vi "Variant to MessagePack Object.vi"(8 "error in (no error)":errorcluster, 11 "Input":variant) -> (0 "error out":errorcluster, 3 "msgpack item":u8[](array[numeric]))   [LabVIEW 2020, in "MessagePack.lvlib"]
uses:
  MessagePack.lvlib
  <vilib>/Utility/Data Type/NI_Data Type.lvlib
  635b5c30-cc5e-43b6-8e2f-470f16c0d6f1.vi
  MsgPackString/MsgPackString.lvclass
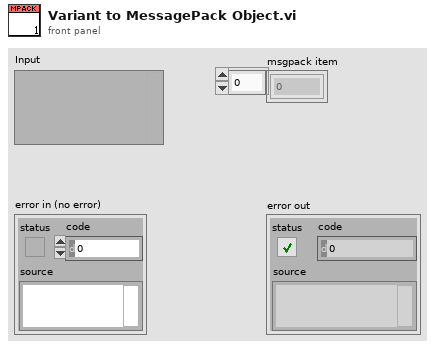
[diagram p1: front panel]
types:
  T1 = typedef "NI_Data Type.lvlib/Data Type.ctl" = enum8{"Invalid Type", "Void", "I8", "I16", "I32", "I64", "U8", "U16", "U32", "U64", "Single Float", "Double Float", "Extended Float", "Single Complex", "Double Complex", "Extended Complex", "Enum U8", "Enum U16", "Enum U32", "Enum U64", "Single Float With Unit", "Double Float With Unit", "Extended Float With Unit", "Single Complex with Unit", "Double Complex with Unit", "Extended Complex with Unit", "Boolean", "String", "Path", "Picture", "Tag", "Array", "Cluster", "Variant", "LV Variant", "Waveform", "Timestamp", "Digital Waveform", "Digital Data", "ExpressData", "Refnum", "External Data", "VI", "Poly VI", "LabVIEW Class Instance", "Fixed Point", "Set Collection", "Map Collection"}
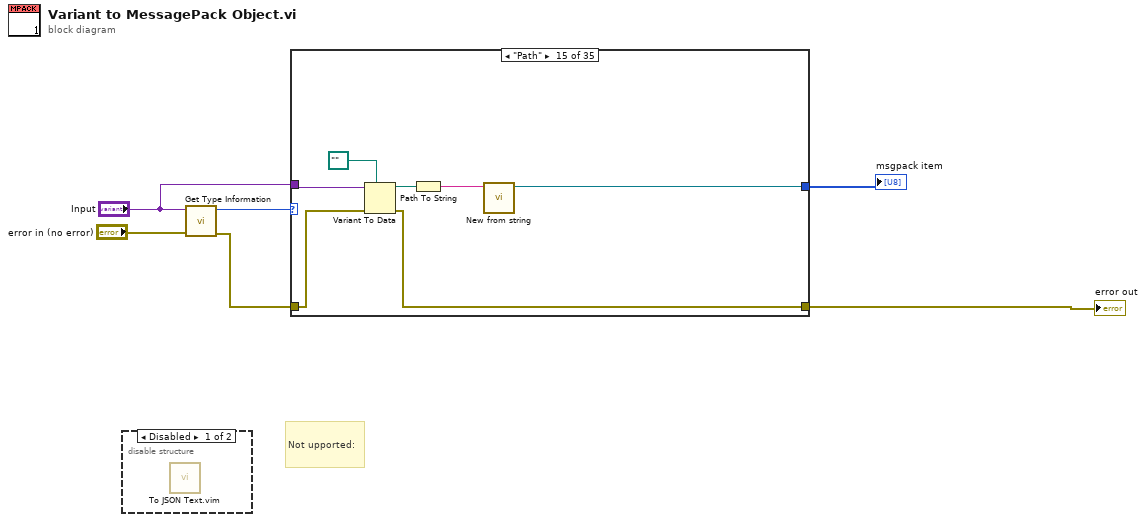
[diagram p0: block diagram]
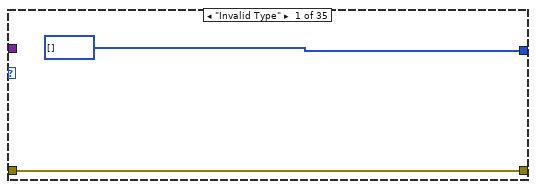
[diagram p3: hidden frame]
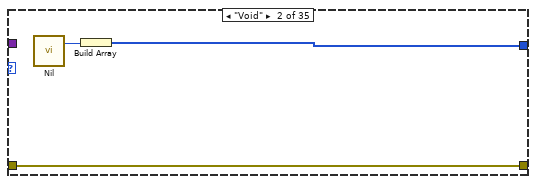
[diagram p4: hidden frame]
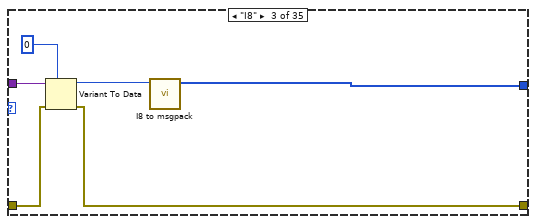
[diagram p5: hidden frame]
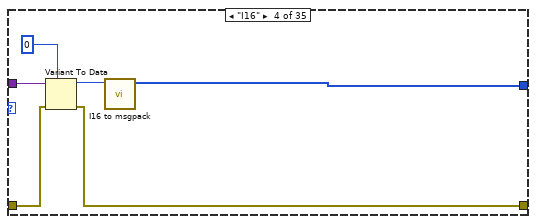
[diagram p6: hidden frame]
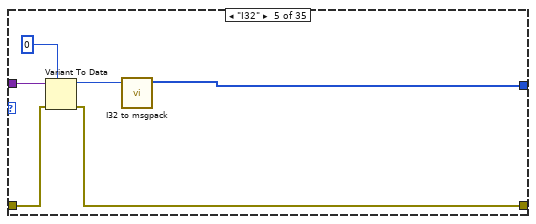
[diagram p7: hidden frame]
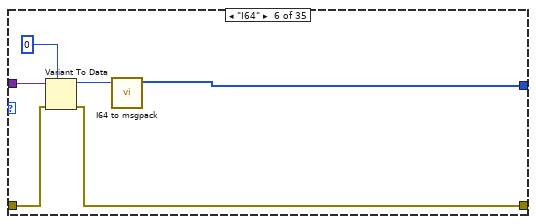
[diagram p8: hidden frame]
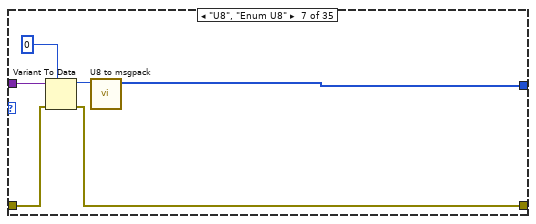
[diagram p9: hidden frame]
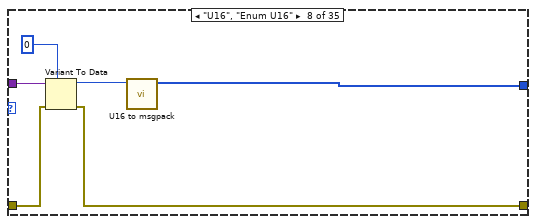
[diagram p10: hidden frame]
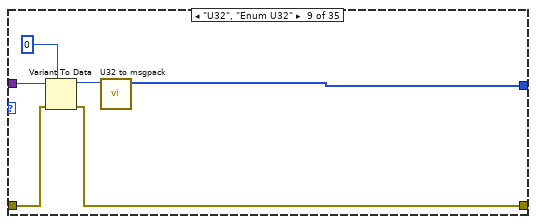
[diagram p11: hidden frame]
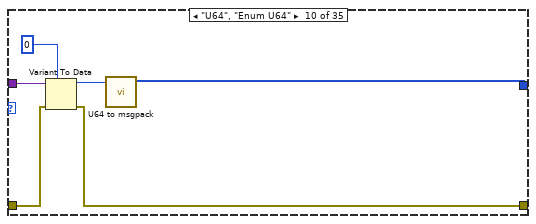
[diagram p12: hidden frame]
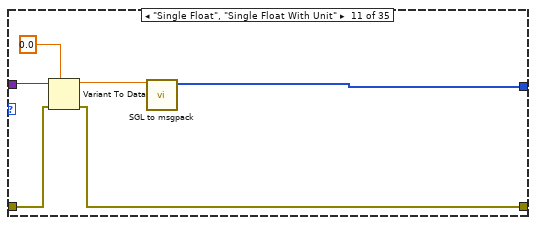
[diagram p13: hidden frame]
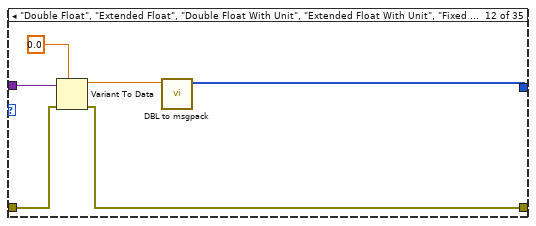
[diagram p14: hidden frame]
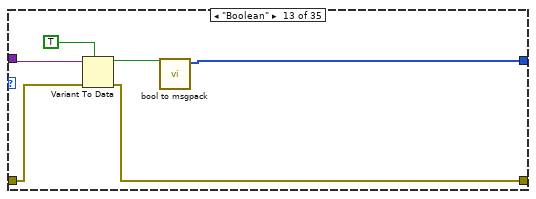
[diagram p15: hidden frame]
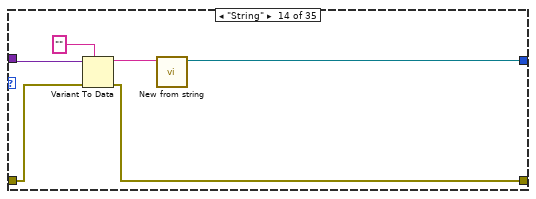
[diagram p16: hidden frame]
diagram:
  # "Not upported:"
  n1 = disable-structure shown="Disabled" {
    frame Disabled {
      n2 = call "To JSON Text.vim"() -> ()  [unwired: 10 in, 2 out]
    }
    frame Enabled {
    }
  }
  n3 = call <vilib>:"Get Type Information.vi"("error in (no error)"="error in (no error)", "variant"="Input") -> ("error out"=w4:errorcluster, "type"=w5:T1)  [unwired: 5 in, 3 out]
  n4 = case shown="\"Path\"" w5 {
    tunnel: w4 -> [w8 w11 w13 w21 w27 w33 w39 w45 w51 w57 w63 w70 w73 w82 w89 _ _ _ _ w96 _ _ _ _ _ _ _ _ _ _ _ _ _ w101 w107]
    tunnel: [w8 w11 w12 w20 w26 w32 w38 w44 w50 w56 w62 w69 w72 w81 w88 _ _ _ _ w91 _ _ _ _ _ _ _ _ _ _ _ _ _ w98 w107] -> w3
    tunnel: [u8[] [] ("msgpack item") w10 w14 w18 w24 w30 w36 w42 w48 w54 w60 w66 w74 w78 w87 _ _ _ _ w92 _ _ _ _ _ _ _ _ _ _ _ _ _ w99 _] -> w2
    tunnel: "Input" -> [_ _ w17 w23 w29 w35 w41 w47 w53 w59 w64 w68 w77 w83 w90 _ _ _ _ w97 _ _ _ _ _ _ _ _ _ _ _ _ _ w102 _]
    frame "Invalid Type" {
    }
    frame "Void" {
      n5 = call "Nil.vi"() -> ("msgpack null"=w9:u8)  [unwired: 7 in]
      n6 = Build Array(w9) -> (w10:u8[])
    }
    frame "I8" {
      n7 = Variant To Data(error in=w13, type=i8 0, Variant=w17) -> (data=w15:i8, error out=w12:errorcluster)
      n8 = call "I8 to msgpack.vi"("I8"=w15) -> ("bytes add"=w14:u8[])  [unwired: 10 in]
    }
    frame "I16" {
      n9 = Variant To Data(error in=w21, type=i16 0, Variant=w23) -> (data=w19:i16, error out=w20:errorcluster)
      n10 = call "I16 to msgpack.vi"("I16"=w19) -> ("bytes add"=w18:u8[])  [unwired: 10 in]
    }
    frame "I32" {
      n11 = Variant To Data(error in=w27, type=0, Variant=w29) -> (data=w25:i32, error out=w26:errorcluster)
      n12 = call "I32 to msgpack.vi"("I32"=w25) -> ("bytes add"=w24:u8[])  [unwired: 10 in]
    }
    frame "I64" {
      n13 = Variant To Data(error in=w33, type=i64 0, Variant=w35) -> (data=w31:i64, error out=w32:errorcluster)
      n14 = call "I64 to msgpack.vi"("I64"=w31) -> ("bytes add"=w30:u8[])  [unwired: 10 in]
    }
    frame "U8", "Enum U8" {
      n15 = Variant To Data(error in=w39, type=u8 0, Variant=w41) -> (data=w37:u8, error out=w38:errorcluster)
      n16 = call "U8 to msgpack.vi"("U8"=w37) -> ("msgpack"=w36:u8[])  [unwired: 10 in]
    }
    frame "U16", "Enum U16" {
      n17 = Variant To Data(error in=w45, type=u16 0, Variant=w47) -> (data=w43:u16, error out=w44:errorcluster)
      n18 = call "U16 to msgpack.vi"("U16"=w43) -> ("msgpack"=w42:u8[])  [unwired: 10 in]
    }
    frame "U32", "Enum U32" {
      n19 = Variant To Data(error in=w51, type=u32 0, Variant=w53) -> (data=w49:u32, error out=w50:errorcluster)
      n20 = call "U32 to msgpack.vi"("U32"=w49) -> ("bytes add"=w48:u8[])  [unwired: 10 in]
    }
    frame "U64", "Enum U64" {
      n21 = Variant To Data(error in=w57, type=u64 0, Variant=w59) -> (data=w55:u64, error out=w56:errorcluster)
      n22 = call "U64 to msgpack.vi"("U64"=w55) -> ("msgpack"=w54:u8[])  [unwired: 10 in]
    }
    frame "Single Float", "Single Float With Unit" {
      n23 = Variant To Data(error in=w63, type=sgl 0.0, Variant=w64) -> (data=w61:sgl, error out=w62:errorcluster)
      n24 = call "SGL to msgpack.vi"("SGL"=w61) -> ("msgpack"=w60:u8[])  [unwired: 10 in]
    }
    frame "Double Float", "Extended Float", "Double Float With Unit", "Extended Float With Unit", "Fixed Point" {
      n25 = Variant To Data(error in=w70, type=0.0, Variant=w68) -> (data=w67:dbl, error out=w69:errorcluster)
      n26 = call "DBL to msgpack.vi"("DBL"=w67) -> ("msgpack"=w66:u8[])  [unwired: 10 in]
    }
    frame "Boolean" {
      n27 = Variant To Data(error in=w73, type=TRUE, Variant=w77) -> (data=w75:bool, error out=w72:errorcluster)
      n28 = call "bool to msgpack.vi"("Boolean"=w75) -> ("msgpack"=w74:u8[])  [unwired: 10 in]
    }
    frame "String" {
      n29 = Variant To Data(error in=w82, type="", Variant=w83) -> (data=w79:string, error out=w81:errorcluster)
      n30 = call "New from string.vi"("String"=w79) -> ("output cluster"=w78:refnum<class "MsgPackString.lvclass">)  [unwired: 10 in]
    }
    frame "Path" {
      n31 = Variant To Data(error in=w89, type=path "", Variant=w90) -> (data=w85:path, error out=w88:errorcluster)
      n32 = Path To String(path=w85) -> (string=w84:string)
      n33 = call "New from string.vi"("String"=w84) -> ("output cluster"=w87:refnum<class "MsgPackString.lvclass">)  [unwired: 10 in]
    }
    frame "Picture" {
    }
    frame "Tag" {
    }
    frame "Array" {
    }
    frame "Cluster" {
    }
    frame "Variant", "LV Variant" {
      n34 = Variant To Data(error in=w96, type=variant, Variant=w97) -> (data=w94:variant, error out=w93:errorcluster)
      n35 = call "Variant to MessagePack Object.vi"("error in (no error)"=w93, "Input"=w94) -> ("error out"=w91:errorcluster, "msgpack item"=w92:u8[])  [unwired: 8 in]
    }
    frame "Waveform" {
    }
    frame "Timestamp" {
    }
    frame "Digital Waveform" {
    }
    frame "Digital Data" {
    }
    frame "ExpressData" {
    }
    frame "Refnum" {
    }
    frame "External Data" {
    }
    frame "VI" {
    }
    frame "Poly VI" {
    }
    frame "LabVIEW Class Instance" {
    }
    frame "Fixed Point" {
    }
    frame "Set Collection" {
    }
    frame "Map Collection" {
    }
    frame "Single Complex".."Extended Complex", "Single Complex with Unit".."Extended Complex with Unit" {
      # "save complex numbers as string"
      n36 = Variant To Data(error in=w101, type=cxt 0.0+0.0i, Variant=w102) -> (data=w105:cxt, error out=w104:errorcluster)
      n37 = Format Into String(format string="%.;%#g", error in=w104, w105) -> (resulting string=w100:string, error out=w98:errorcluster)  [unwired: 1 in]
      n38 = call "New from string.vi"("String"=w100) -> ("output cluster"=w99:refnum<class "MsgPackString.lvclass">)  [unwired: 10 in]
    }
    frame Default {
    }
  }
  "msgpack item" <- w2
  "error out" <- w3
